vi "Create Motor.vi"(0 "reference in":refnum<class "EngineFactory.lvclass">, 11 "Error In":errorcluster) -> (4 "reference out":refnum<class "EngineFactory.lvclass">, 6 "IMotor":refnum<class "IMotor.lvclass">, 15 "Error Out":errorcluster)   [LabVIEW 2024, in "EngineFactory.lvclass"]
uses:
  EngineFactory.lvclass
  EngineFactory.lvclass/EngineFactory.ctl
  Product Folder/IMotor/IMotor.lvclass
panel:
  # "Connector Pane"
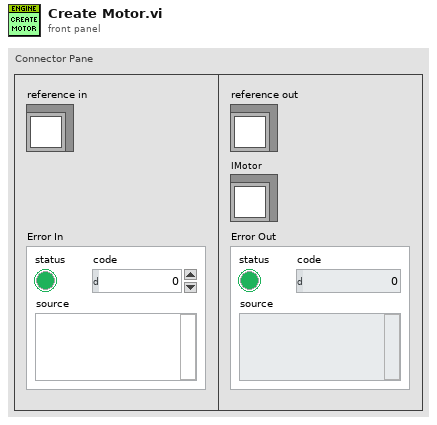
[diagram p1: front panel]
types:
  T1 = typedef "EngineFactory.lvclass/ObjectAttributes.ctl" = cluster{"None":bool}
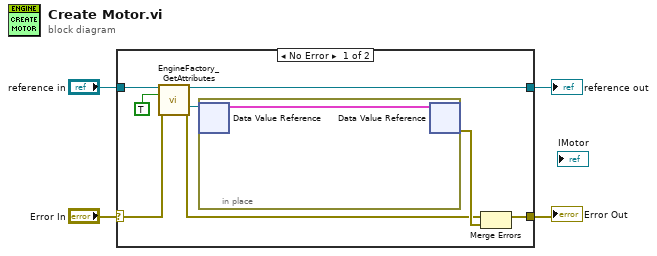
[diagram p0: block diagram]
diagram:
  n1 = case shown="No Error" "Error In" {
    selector: "Error In" -> [w11 w15]
    tunnel: [w8 w15] -> w3
    tunnel: [w9 w14] -> w1
    tunnel: "reference in" -> [w12 w14]
    frame No Error {
      n2 = call "EngineFactory_GetAttributes.vi"("reference in"=w12, "OnlyGetDvrReference(False)"=TRUE, "Error In"=w11) -> ("reference out"=w9:refnum<class "EngineFactory.lvclass">, "DataRef"=w7:refnum<data-value>, "Error Out"=w6:errorcluster)  [unwired: 9 in, 1 out]
      n3 = in-place {
        n4 = in-place-dvr #1(w7) -> (w13:T1)  [unwired: 1 out]
        n5 = in-place-dvr #1(w13) -> (w10:errorcluster)  [unwired: 1 out]
      }
      n6 = Merge Errors(w6, w10) -> (w8:errorcluster)
    }
    frame Error {
    }
  }
  "Error Out" <- w3
  "reference out" <- w1
